vi "create.TradeShort.vi"(8 "error in (no error)":errorcluster, 11 "TradeShort.Parmeters":T1={"Time Offset"=447000, "Order Id"="ORID0001", "Execution Id"="EXE_ID_1", "Quantity"=20000, "Price"=0.905, "Side Indicator"="B", "Symbol"="AAPL"}) -> (0 "error out":errorcluster, 2 "Bytes.out":u8[](array[numeric]) format="%.0x", 3 "MessageBase out":refnum<class "TradeShort.lvclass">)   [LabVIEW 2022 SP3]
uses:
  Trade/TradeShort.Parameters.ctl
  Trade/TradeShort.lvclass
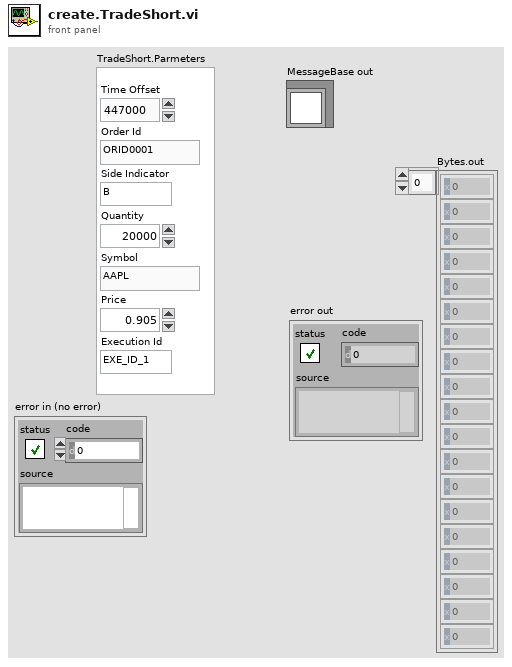
[diagram p1: front panel]
types:
  T1 = typedef "TradeShort.lvclass/TradeShort.Parameters.ctl" = cluster{"Time Offset":u32, "Order Id":string, "Execution Id":string, "Quantity":u32, "Price":dbl, "Side Indicator":string, "Symbol":string}
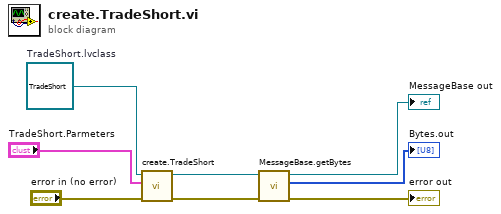
[diagram p0: block diagram]
diagram:
  w5 = refnum<class "TradeShort.lvclass"> refnum  # TradeShort.lvclass
  n1 = call-dynamic "create.TradeShort.vi"("error in"="error in (no error)", "TradeShort.Parameters"="TradeShort.Parmeters", "TradeShort in"=w5) -> ("error out"=w3:errorcluster, "TradeShort out"=w2:refnum<class "TradeShort.lvclass">)  [unwired: 7 in]
  n2 = call-dynamic "MessageBase.getBytes.vi"("error in (no error)"=w3, "MessageBase in"=w2) -> ("error out"=→"error out":errorcluster, "Bytes.out"=→"Bytes.out":u8[], "MessageBase out"=→"MessageBase out":refnum<class "TradeShort.lvclass">)  [unwired: 7 in]
